vi "4 probe data-osc-keith v1.4.vi"() -> ()   [LabVIEW 2014]
uses:
  <vilib>/Analysis/baseanly.llb/Mean (DBL).vi
  <instrlib>/Keithley 24XX/Public/Data/Read (Single Point).vi
  <instrlib>/Tektronix TDS 200 1000 2000 Series/Tektronix TDS 200 1000 2000 Series.lvlib
  <vilib>/Analysis/NI_AALBase.lvlib
  <instrlib>/Keithley 24XX/Keithley 24XX.lvlib
panel:
  out "Resistance-Time":sgl[](graph)
  out "Data IV Keithley":string
  in  "Data IV Keithley 2":path=path "c:/myfile.txt"
  out "IV Curve":cluster{sgl[], dbl[]}(graph)
  in  "Stop Voltage/Current":dbl=2.0
  in  "VISA resource name 2":refnum<visa-resource-name>="GPIB9::24::INSTR"
  in  "Serial Configuration 2":T1={"Baud Rate"=9600, "Parity"=0, "Data Bits"=8, "Stop Bits"=10, "Flow Control"=0} {"Flow Control" items=["None", "XON/XOFF", "RTS/CTS", "XON/XOFF & RTS/CTS", "DTR/DSR", "XON/XOFF & DTR/DSR"]; "Stop Bits" items=["1.0"=10, "1.5"=15, "2.0"=20]; "Data Bits" items=["7"=7, "8"=8]; "Parity" items=["None", "Odd", "Even", "Mark", "Space"]; "Baud Rate" items=["300"=300, "600"=600, "1200"=1200, "2400"=2400, "4800"=4800, "9600"=9600, "19200"=19200]}
  out "Voltage":sgl
  out "Current":sgl
  out "Resistance":sgl
  in  "Voltage Manual Range (1.0)":dbl=1.0
  in  "Current Manual Range (1.0)":dbl=1.0
  in  "Resistance Manual Range (1.0)":dbl=1.0
  in  "Enable Voltage Auto Range (T:Enable)":bool
  in  "Enable Current Auto Range (T:Enable)":bool=TRUE
  in  "Enable Resistance Auto Range (T:Enable)":bool
  in  "Compliance  Level (0.1)":dbl=1.0
  in  "Source Mode  (0: Voltage)":u16(ring) items=["Voltage", "Current"]
  in  "Step":dbl=1.0
  in  "current multiplier":dbl=1.0
  in  "Start Voltage/Current":dbl
  in  "Stop Button":bool
  out "Data Ch4":string
  in  "Data Ch4":path=path "c:/myfile4.txt"
  out "Ard3-Osc4":cluster{"Y":dbl[], "Y":dbl[]}[](graph)
  out "Ch1":dbl
  out "Ch2":dbl
  out "Ch3":dbl
  out "Ch4":dbl
  in  "Channel 4 (3: Channel 4)":u16(ring)=3 items=["Channel 1", "Channel 2", "Channel 3", "Channel 4", "Math", "Reference A", "Reference B", "Reference C", "Reference D"]
  in  "Probe Attenuation 4 (0.1)":dbl=0.1
  in  "Vertical Coupling 4 (1: DC)":u16(ring)=1 items=["AC", "DC", "Ground"]
  in  "Channel 3 (2: Channel 3)":u16(ring)=2 items=["Channel 1", "Channel 2", "Channel 3", "Channel 4", "Math", "Reference A", "Reference B", "Reference C", "Reference D"]
  in  "Probe Attenuation 3 (0.1)":dbl=0.1
  in  "Vertical Coupling 3 (1: DC)":u16(ring)=1 items=["AC", "DC", "Ground"]
  in  "Channel 2 (1: Channel 2)":u16(ring)=1 items=["Channel 1", "Channel 2", "Channel 3", "Channel 4", "Math", "Reference A", "Reference B", "Reference C", "Reference D"]
  in  "Channel 1 (0: Channel 1)":u16(ring) items=["Channel 1", "Channel 2", "Channel 3", "Channel 4", "Math", "Reference A", "Reference B", "Reference C", "Reference D"]
  in  "Serial Configuration":T2={"Baud Rate"=9600, "Parity"=0, "Stop Bits"=10, "Flow Control"=2} {"Flow Control" items=["None", "XON/XOFF", "RTS/CTS", "XON/XOFF & RTS/CTS", "DTR/DSR", "XON/XOFF & DTR/DSR"]; "Stop Bits" items=["1.0"=10, "1.5"=15, "2.0"=20]; "Parity" items=["None", "Odd", "Even", "Mark", "Space"]; "Baud Rate" items=["300"=300, "600"=600, "1200"=1200, "2400"=2400, "4800"=4800, "9600"=9600, "19200"=19200]}
  in  "Probe Attenuation 2 (0.1)":dbl=0.1
  in  "Vertical Coupling 2 (1: DC)":u16(ring)=1 items=["AC", "DC", "Ground"]
  in  "Probe Attenuation 1 (0.1)":dbl=0.1
  in  "Vertical Coupling 1 (1: DC)":u16(ring)=1 items=["AC", "DC", "Ground"]
  in  "Timeout (10000 ms)":u32=500
  in  "VISA resource name":refnum<visa-resource-name>="USB0::0x0699::0x03A6::C044157::INSTR"
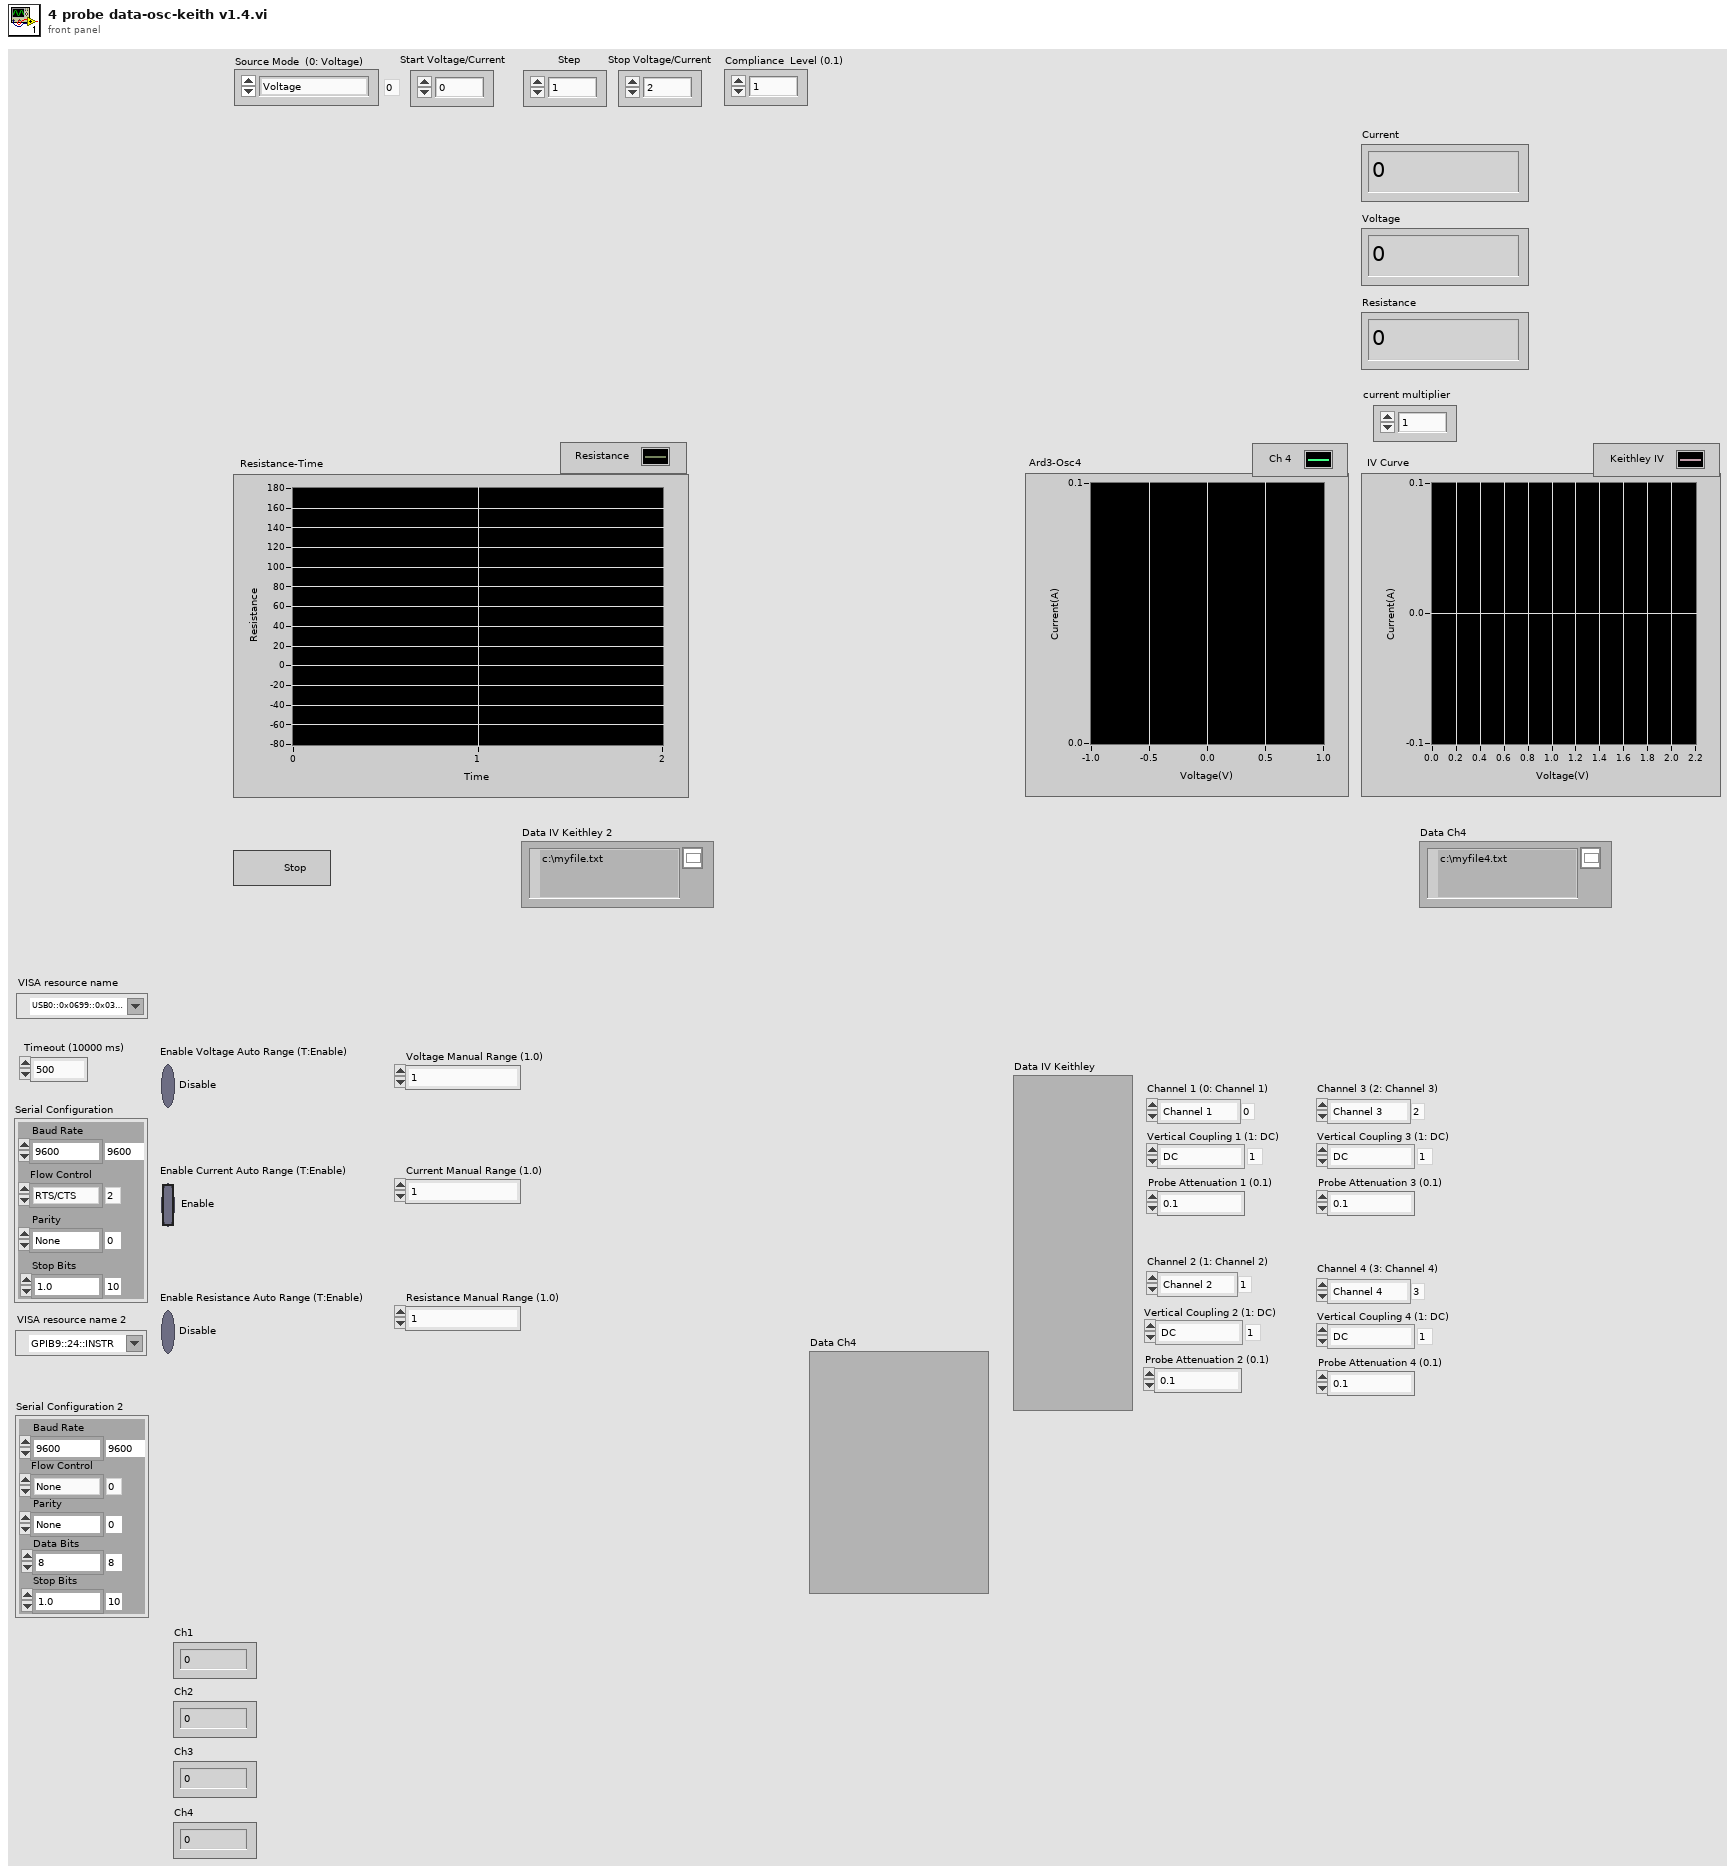
[diagram p1: front panel]
types:
  T1 = cluster{"Baud Rate":u32, "Parity":u16, "Data Bits":u16, "Stop Bits":u16, "Flow Control":u16}
  T2 = cluster{"Baud Rate":u32, "Parity":u16, "Stop Bits":u16, "Flow Control":u16}
  T3 = enum16{"open", "replace", "create", "open or create", "replace or create", "replace or create with confirmation"}
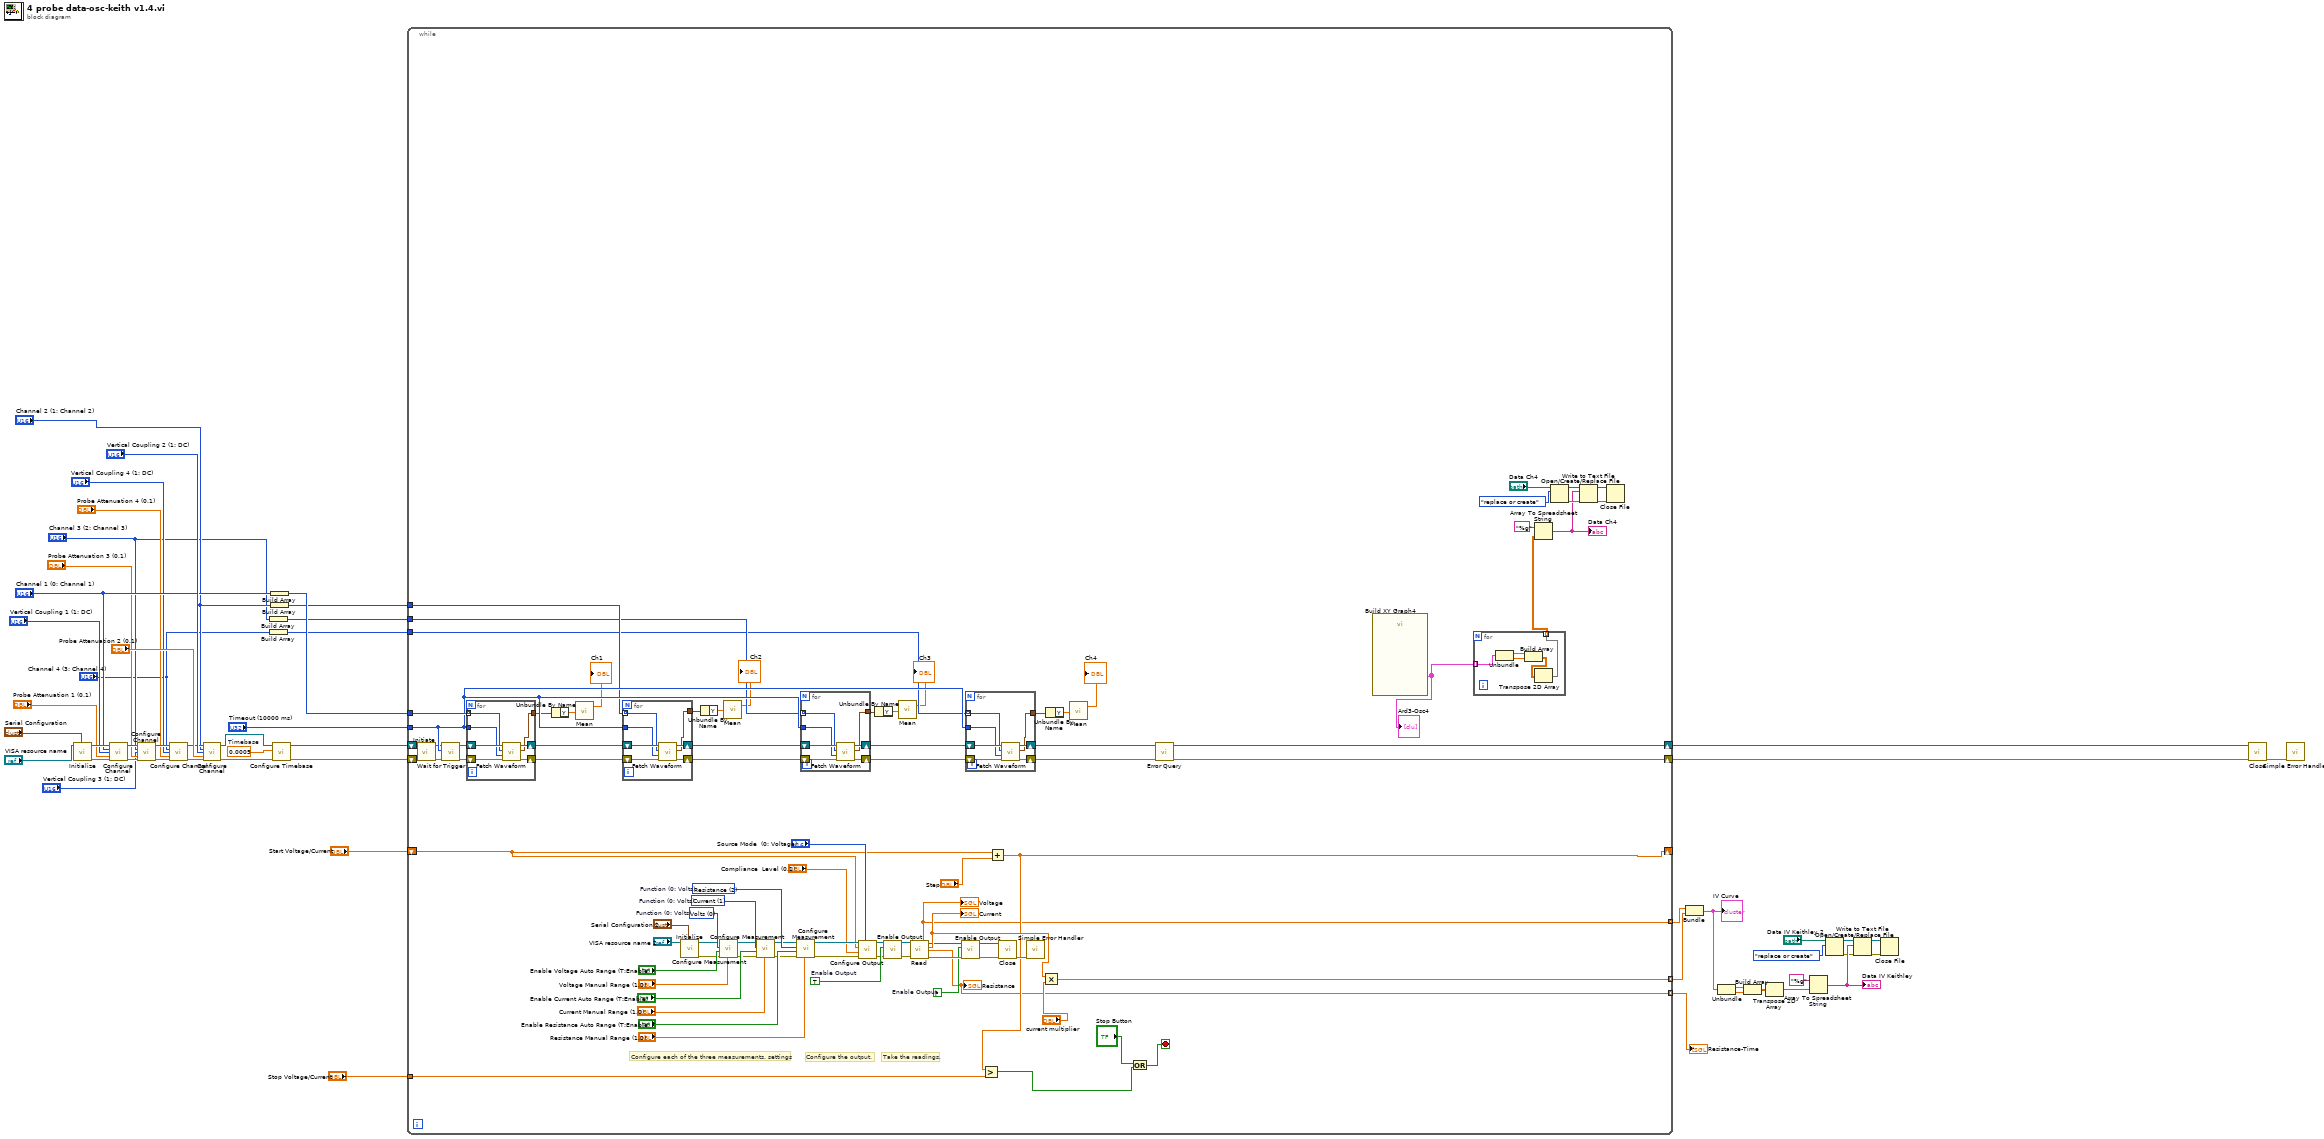
[diagram p0: block diagram]
diagram:
  w39 = 0.0005  # Timebase
  n1 = call <instrlib>:"Initialize.vi"("Serial Configuration"="Serial Configuration", "VISA resource name"="VISA resource name") -> ("error out"=w48:errorcluster, "VISA resource name out"=w49:refnum<visa-resource-name>)  [unwired: 3 in, 5 out]
  n2 = call <instrlib>:"Configure Channel.vi"("VISA resource name"=w49, "Channel (0: Channel 1)"="Channel 1 (0: Channel 1)", "Vertical Coupling (1: DC)"="Vertical Coupling 1 (1: DC)", "Probe Attenuation (10: 10X)"="Probe Attenuation 1 (0.1)", "error in (no error)"=w48) -> ("VISA resource name out"=w34:refnum<visa-resource-name>, "error out"=w31:errorcluster)  [unwired: 4 in, 5 out]
  n3 = call <instrlib>:"Configure Channel.vi"("VISA resource name"=w34, "Channel (0: Channel 1)"="Channel 3 (2: Channel 3)", "Vertical Coupling (1: DC)"="Vertical Coupling 3 (1: DC)", "Probe Attenuation (10: 10X)"="Probe Attenuation 3 (0.1)", "error in (no error)"=w31) -> ("VISA resource name out"=w33:refnum<visa-resource-name>, "error out"=w30:errorcluster)  [unwired: 4 in, 5 out]
  n4 = call <instrlib>:"Configure Channel.vi"("VISA resource name"=w33, "Channel (0: Channel 1)"="Channel 4 (3: Channel 4)", "Vertical Coupling (1: DC)"="Vertical Coupling 4 (1: DC)", "Probe Attenuation (10: 10X)"="Probe Attenuation 4 (0.1)", "error in (no error)"=w30) -> ("VISA resource name out"=w32:refnum<visa-resource-name>, "error out"=w29:errorcluster)  [unwired: 4 in, 5 out]
  n5 = call <instrlib>:"Configure Channel.vi"("VISA resource name"=w32, "Channel (0: Channel 1)"="Channel 2 (1: Channel 2)", "Vertical Coupling (1: DC)"="Vertical Coupling 2 (1: DC)", "Probe Attenuation (10: 10X)"="Probe Attenuation 2 (0.1)", "error in (no error)"=w29) -> ("VISA resource name out"=w47:refnum<visa-resource-name>, "error out"=w46:errorcluster)  [unwired: 4 in, 5 out]
  n6 = Build Array("Channel 3 (2: Channel 3)") -> (w20:u16[])
  n7 = Build Array("Channel 4 (3: Channel 4)") -> (w19:u16[])
  n8 = Build Array("Channel 1 (0: Channel 1)") -> (w38:u16[])
  n9 = Build Array("Channel 2 (1: Channel 2)") -> (w23:u16[])
  n10 = call <instrlib>:"Configure Timebase.vi"("error in (no error)"=w46, "Timebase (0.0005 s)"=w39, "VISA resource name"=w47) -> ("error out"=w44:errorcluster, "VISA resource name out"=w45:refnum<visa-resource-name>)  [unwired: 1 in, 6 out]
  n11 = while {
    tunnel: w38 -> [w136]
    tunnel: "Timeout (10000 ms)" -> [w135]
    tunnel: w23 -> [w134]
    tunnel: w20 -> [w133]
    tunnel: w19 -> [w132]
    shift-right: [w140] -> w51
    shift-left: w45 -> [w138]
    shift-right: [w139] -> w50
    shift-left: w44 -> [w137]
    tunnel: "Stop Voltage/Current" -> [w62]
    shift-right: [w60] -> _
    shift-left: "Start Voltage/Current" -> [w61]
    tunnel: [w56] -> w3 mode=indexing
    tunnel: [w55] -> w2 mode=indexing
    tunnel: [w54] -> w1 mode=indexing
    stop <- w57 stop-if-true
    w91 = TRUE  # Enable Output
    w81 = FALSE  # Enable Output
    w74 = u16 2 items=["Volts", "Current", "Resistance"]  # Function (0: Volts)
    w73 = u16 1 items=["Volts", "Current", "Resistance"]  # Function (0: Volts)
    w72 = u16 0 items=["Volts", "Current", "Resistance"]  # Function (0: Volts)
    # "Take the readings."
    # "Configure the output."
    # "Configure each of the three measurements. settings"
    n12 = call <instrlib>:"Initiate.vi"("error in (no error)"=w137, "VISA resource name"=w138) -> ("error out"=w128:errorcluster, "VISA resource name out"=w131:refnum<visa-resource-name>)  [unwired: 8 out]
    n13 = call <instrlib>:"Wait for Trigger.vi"("error in (no error)"=w128, "Timeout (10000 ms)"=w135, "VISA resource name"=w131) -> ("error out"=w129:errorcluster, "VISA resource name out"=w130:refnum<visa-resource-name>)  [unwired: 7 out]
    n14 = for {
      shift-right: [w172] -> w126
      shift-left: w129 -> [w170]
      tunnel: w136 -> [w168] mode=indexing
      tunnel: w135 -> [w169]
      shift-right: [w173] -> w127
      shift-left: w130 -> [w171]
      tunnel: [w167] -> w119
      n15 = call <instrlib>:"Fetch Waveform.vi"("error in (no error)"=w170, "Timeout (10000 ms)"=w169, "Source (0: Channel 1)"=w168, "VISA resource name"=w171) -> ("error out"=w172:errorcluster, "Waveform Data"=w167:waveform(dbl), "VISA resource name out"=w173:refnum<visa-resource-name>)  [unwired: 2 in, 3 out]
    }
    n16 = Unbundle By Name(w119) -> ("Y"=w118:dbl[])
    n17 = call-poly <vilib>:"Mean.vi"("X"=w118) -> ("mean"=→"Ch1":dbl)  [unwired: 1 out]
    n18 = for {
      shift-right: [w165] -> w120
      shift-left: w126 -> [w163]
      tunnel: w134 -> [w161] mode=indexing
      tunnel: w135 -> [w162]
      shift-right: [w166] -> w121
      shift-left: w127 -> [w164]
      tunnel: [w160] -> w115
      n19 = call <instrlib>:"Fetch Waveform.vi"("error in (no error)"=w163, "Timeout (10000 ms)"=w162, "Source (0: Channel 1)"=w161, "VISA resource name"=w164) -> ("error out"=w165:errorcluster, "Waveform Data"=w160:waveform(dbl), "VISA resource name out"=w166:refnum<visa-resource-name>)  [unwired: 2 in, 3 out]
    }
    n20 = call <instrlib>:"Initialize.vi"("Serial Configuration"="Serial Configuration 2", "VISA resource name"="VISA resource name 2") -> ("error out"=w67:errorcluster, "VISA resource name out"=w66:refnum<visa-resource-name>)  [unwired: 8 in]
    n21 = Unbundle By Name(w115) -> ("Y"=w114:dbl[])
    n22 = call <instrlib>:"Configure Measurement.vi"("Manual Range (1.0)"="Voltage Manual Range (1.0)", "error in (no error)"=w67, "Enable Auto Range (T:Enable)"="Enable Voltage Auto Range (T:Enable)", "Function (0: Volts)"=w72, "VISA resource name"=w66) -> ("error out"=w69:errorcluster, "VISA resource name out"=w68:refnum<visa-resource-name>)  [unwired: 5 in]
    n23 = call-poly <vilib>:"Mean.vi"("X"=w114) -> ("mean"=→"Ch2":dbl)  [unwired: 1 out]
    n24 = call <instrlib>:"Configure Measurement.vi"("Manual Range (1.0)"="Current Manual Range (1.0)", "error in (no error)"=w69, "Enable Auto Range (T:Enable)"="Enable Current Auto Range (T:Enable)", "Function (0: Volts)"=w73, "VISA resource name"=w68) -> ("error out"=w70:errorcluster, "VISA resource name out"=w71:refnum<visa-resource-name>)  [unwired: 5 in]
    n25 = call <instrlib>:"Configure Measurement.vi"("Manual Range (1.0)"="Resistance Manual Range (1.0)", "error in (no error)"=w70, "Enable Auto Range (T:Enable)"="Enable Resistance Auto Range (T:Enable)", "Function (0: Volts)"=w74, "VISA resource name"=w71) -> ("error out"=w92:errorcluster, "VISA resource name out"=w93:refnum<visa-resource-name>)  [unwired: 5 in]
    n26 = for {
      shift-right: [w158] -> w124
      shift-left: w120 -> [w156]
      tunnel: w133 -> [w154] mode=indexing
      tunnel: w135 -> [w155]
      shift-right: [w159] -> w125
      shift-left: w121 -> [w157]
      tunnel: [w153] -> w116
      n27 = call <instrlib>:"Fetch Waveform.vi"("error in (no error)"=w156, "Timeout (10000 ms)"=w155, "Source (0: Channel 1)"=w154, "VISA resource name"=w157) -> ("error out"=w158:errorcluster, "Waveform Data"=w153:waveform(dbl), "VISA resource name out"=w159:refnum<visa-resource-name>)  [unwired: 2 in, 3 out]
    }
    n28 = call <instrlib>:"Configure Output.vi"("Source Mode  (0: Voltage)"="Source Mode  (0: Voltage)", "error in (no error)"=w92, "Compliance  Level (0.1)"="Compliance  Level (0.1)", "Output Level (0)"=w61, "VISA resource name"=w93) -> ("error out"=w90:errorcluster, "VISA resource name out"=w89:refnum<visa-resource-name>)  [unwired: 5 in]
    n29 = Unbundle By Name(w116) -> ("Y"=w113:dbl[])
    n30 = call <instrlib>:"Enable Output.vi"("error in (no error)"=w90, "Enable Output (T: Enable)"=w91, "VISA resource name"=w89) -> ("error out"=w87:errorcluster, "VISA resource name out"=w88:refnum<visa-resource-name>)  [unwired: 7 in]
    n31 = call-poly <vilib>:"Mean.vi"("X"=w113) -> ("mean"=→"Ch3":dbl)  [unwired: 1 out]
    n32 = call-poly <instrlib>:"Read.vi"("VISA resource name"=w88, "error in (no error)"=w87) -> ("Voltage"=w55:sgl, "VISA resource name out"=w86:refnum<visa-resource-name>, "Current"=w96:sgl, "Resistance"=w54:sgl, "error out"=w85:errorcluster)  [unwired: 7 in, 2 out]
    "Voltage" <- w55
    "Current" <- w96
    "Resistance" <- w54
    n33 = call <instrlib>:"Enable Output.vi"("error in (no error)"=w85, "Enable Output (T: Enable)"=w81, "VISA resource name"=w86) -> ("error out"=w84:errorcluster, "VISA resource name out"=w83:refnum<visa-resource-name>)  [unwired: 7 in]
    n34 = for {
      shift-right: [w151] -> w122
      shift-left: w124 -> [w149]
      tunnel: w132 -> [w147] mode=indexing
      tunnel: w135 -> [w148]
      shift-right: [w152] -> w123
      shift-left: w125 -> [w150]
      tunnel: [w146] -> w117
      n35 = call <instrlib>:"Fetch Waveform.vi"("error in (no error)"=w149, "Timeout (10000 ms)"=w148, "Source (0: Channel 1)"=w147, "VISA resource name"=w150) -> ("error out"=w151:errorcluster, "Waveform Data"=w146:waveform(dbl), "VISA resource name out"=w152:refnum<visa-resource-name>)  [unwired: 2 in, 3 out]
    }
    n36 = Add(x=w61, y="Step") -> (x+y=w60:dbl)
    n37 = Greater?(x=w60, y=w62) -> (0:w59:bool)
    n38 = call <instrlib>:"Close.vi"("error in (no error)"=w84, "VISA resource name"=w83) -> ("error out"=w63:errorcluster)  [unwired: 9 in]
    n39 = call <vilib>:"Simple Error Handler.vi"("error in (no error)"=w63) -> ()  [unwired: 4 in, 5 out]
    n40 = Multiply(x=w96, y="current multiplier") -> (x*y=w56:dbl)
    n41 = Unbundle By Name(w117) -> ("Y"=w112:dbl[])
    n42 = call-poly <vilib>:"Mean.vi"("X"=w112) -> ("mean"=→"Ch4":dbl)  [unwired: 1 out]
    n43 = Or(x="Stop Button", y=w59) -> (x .or. y?=w57:bool)
    n44 = call <instrlib>:"Error Query.vi"("error in (no error)"=w122, "VISA resource name"=w123) -> ("error out"=w139:errorcluster, "VISA resource name out"=w140:refnum<visa-resource-name>)  [unwired: 8 out]
    n45 = call "Build XY Graph4"() -> ("XY Graph"=w99:cluster{"Y":dbl[], "Y":dbl[]}[])  [unwired: 10 in, 1 out]
    "Ard3-Osc4" <- w99
    n46 = for {
      tunnel: w99 -> [w145] mode=indexing
      tunnel: [w141] -> w100 mode=indexing
      n47 = Unbundle(w145) -> ("Y"=w144:dbl[], "Y"=w143:dbl[])
      n48 = Build Array(w144, w143) -> (w142:dbl[][])
      n49 = Transpose 2D Array(2D array=w142) -> (transposed array=w141:dbl[][])
    }
    n50 = Array To Spreadsheet String(array=w100, 3:"%g" ("format string")) -> (spreadsheet string=w101:string)  [unwired: 1 in]
    "Data Ch4" <- w101
    n51 = Open/Create/Replace File(file path (use dialog)="Data Ch4", operation (0:open)=T3."replace or create") -> (refnum out=w103:refnum<file>, error out=w108:errorcluster)  [unwired: 4 in, 1 out]
    n52 = Write to Text File(file (use dialog)=w103, text=w101, error in=w108) -> (refnum out=w106:refnum<file>, error out=w107:errorcluster)  [unwired: 2 out]
    n53 = Close File(refnum=w106, error in=w107) -> ()  [unwired: 2 out]
  }
  "Resistance-Time" <- w1
  n54 = Bundle(w2, w3) -> (w12:cluster{sgl[], dbl[]})  [unwired: 1 out]
  "IV Curve" <- w12
  n55 = Unbundle(w12) -> (w13:sgl[], w14:dbl[])
  n56 = Build Array(w13, w14) -> (w15:dbl[][])
  n57 = Transpose 2D Array(2D array=w15) -> (transposed array=w17:dbl[][])
  n58 = Array To Spreadsheet String(array=w17, 3:"%g" ("format string")) -> (spreadsheet string=w18:string)  [unwired: 1 in]
  "Data IV Keithley" <- w18
  n59 = Open/Create/Replace File(file path (use dialog)="Data IV Keithley 2", operation (0:open)=T3."replace or create") -> (refnum out=w11:refnum<file>, error out=w6:errorcluster)  [unwired: 4 in, 1 out]
  n60 = Write to Text File(file (use dialog)=w11, text=w18, error in=w6) -> (refnum out=w8:refnum<file>, error out=w7:errorcluster)  [unwired: 2 out]
  n61 = Close File(refnum=w8, error in=w7) -> ()  [unwired: 2 out]
  n62 = call <instrlib>:"Close.vi"("error in (no error)"=w50, "VISA resource name"=w51) -> ("error out"=w52:errorcluster)  [unwired: 9 out]
  n63 = call <vilib>:"Simple Error Handler.vi"("error in (no error)"=w52) -> ()  [unwired: 1 in, 8 out]
